vi "Autonomous Independent.vi"() -> ()   [LabVIEW 2019]
doc: "This VI is called when autonomous begins, and will automatically be terminated when autonomous ends. You can carry out timed or sensor driven robot movement independently without needing to return to the caller."
uses:
  <vilib>/Rock Robotics/SystemInterfaces/spilib/spi_bus.ctl
  <vilib>/Rock Robotics/WPI/Utilities/WPI_GetSetVariantRefNum.vi
  <vilib>/Rock Robotics/Network Tables/NT Write Numeric Array.vi
  <vilib>/Rock Robotics/WPI/RobotDrive/WPI_RobotDriveArcadeDrive_Standard(NoSaturation).vi
  <vilib>/Rock Robotics/WPI/Gyro/WPI_GyroXRS450_SPI_Open.vi
  <vilib>/Rock Robotics/Network Tables/NT Write Number.vi
  <vilib>/Rock Robotics/Network Tables/NT Read String.vi
panel:
  out "Ultrasonic 2":dbl
  out "Ultrasonic":dbl
  out "Degrees 2":dbl(knob) scale=0.0..360.0
  out "Degrees":dbl(knob) scale=0.0..360.0
  in  "Reset Angle?":bool
  out "Calibrated?":bool
  out "Degrees":dbl(knob) scale=0.0..360.0
  out "Degrees 2":dbl(knob) scale=0.0..360.0
  in  "SPI Bus":T1
  out "Device Found":bool
  in  "Sample Rate (Hz)":dbl=1000.0 min=50.0 max=20000.0 format="%#_13g"
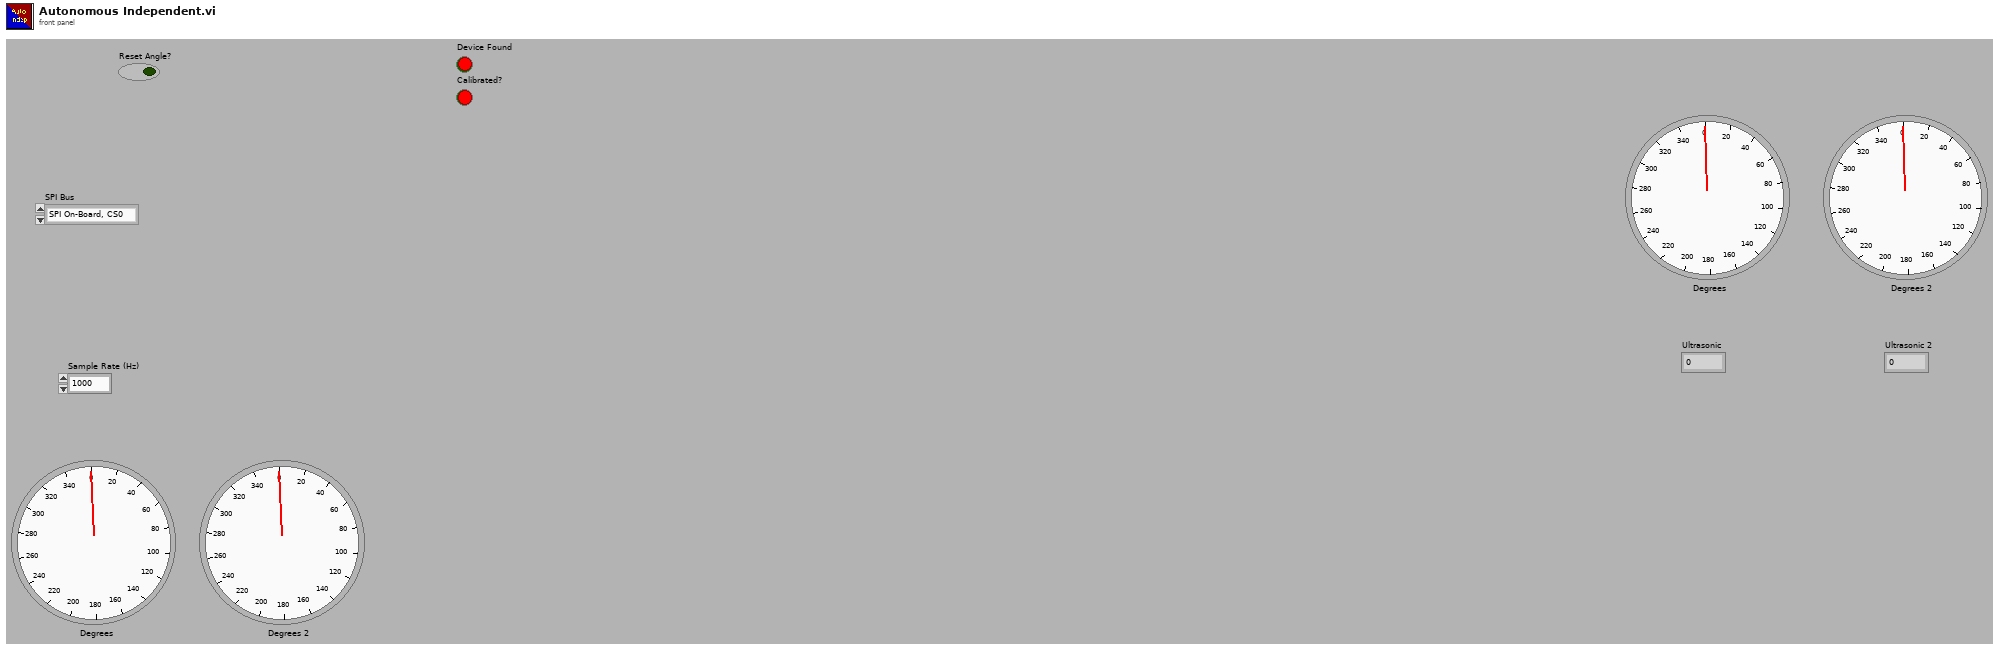
[diagram p1: front panel]
types:
  T1 = typedef "spi_bus.ctl" = enum16{"SPI On-Board, CS0", "SPI On-Board, CS1", "SPI On-Board, CS2", "SPI On-Board, CS3", "SPI MXP", "Invalid"}
  T2 = typedef "WPI_JoystickDevRef.ctl" = cluster{"Device":T3}
  T3 = typedef "WPI_JoystickDeviceEnum.ctl" = enum16{"USB 0", "USB 1", "USB 2", "USB 3", "USB 4", "USB 5"}
  T4 = typedef "WPI_RobotDriveDevRef.ctl" = cluster{"DevStatus":errorcluster, "Motors[]":T5[], "Square Inputs":bool, "Max Output":dbl}
  T5 = typedef "WPI_MotorControlDeviceRef.ctl" = cluster{"DeviceStatus":errorcluster, "Type":T6, "PWM":cluster{"PWM Channel":T7, "DeadBand":T8}, "CAN":cluster{"Device Number":u8, "SetOutput VI Ref":variant, "GetOutput VI Ref":variant, "Enable VI Ref":variant, "Disable VI Ref":variant, "Data":variant}, "Invert":bool, "DIO PWM":cluster{"PWM \"Enable\" Channel":T7, "DIOChannel":T9, "PWM Rate":dbl}}
  T6 = typedef "WPI_MotorControlType.ctl" = enum16{"PWM", "CAN", "DIO PWM"}
  T7 = typedef "FPGA_DIOPWMChannel.ctl" = enum8{"PWM 0", "PWM 1", "PWM 2", "PWM 3", "PWM 4", "PWM 5", "PWM 6", "PWM 7", "PWM 8", "PWM 9", "PWM MXP 0", "PWM MXP 1", "PWM MXP 2", "PWM MXP 3", "PWM MXP 4", "PWM MXP 5", "PWM MXP 6", "PWM MXP 7", "PWM MXP 8", "PWM MXP 9", "Invalid"}
  T8 = typedef "WPI_PWMDeadband.ctl" = cluster{"Name":string, "maxPositivePwm":i32, "minPositivePwm":i32, "centerPwm":i32, "maxNegativePwm":i32, "minNegativePwm":i32, "angularRange":u16}
  T9 = typedef "FPGA_DIOChannel.ctl" = enum8{"DIO 0", "DIO 1", "DIO 2", "DIO 3", "DIO 4", "DIO 5", "DIO 6", "DIO 7", "DIO 8", "DIO 9", "DIO MXP 0", "DIO MXP 1", "DIO MXP 2", "DIO MXP 3", "DIO MXP 4", "DIO MXP 5", "DIO MXP 6", "DIO MXP 7", "DIO MXP 8", "DIO MXP 9", "DIO MXP 10", "DIO MXP 11", "DIO MXP 12", "DIO MXP 13", "DIO MXP 14", "DIO MXP 15", "SPI Port CS1", "SPI Port CS2", "SPI Port CS3", "SPI Port MISO", "SPI Port MOSI", "Invalid"}
  T10 = typedef "WPI_GyroDevRef.ctl" = cluster{"DevStatus":errorcluster, "Analog Channel":T11, "Gain (VoltsPerDegree/Second)":dbl, "Gyro Type":enum16{"Analog", "XRS450"}, "Handle":i32, "SPI Bus":T1, "Device Found":bool, "Sample Rate":dbl, "Calibrate On Open":bool, "Offset":dbl}
  T11 = typedef "FPGA_AIChannel.ctl" = enum8{"AI 0", "AI 1", "AI 2", "AI 3", "AI MXP 0", "AI MXP 1", "AI MXP 2", "AI MXP 3", "Invalid"}
  T12 = typedef "WPI_AnalogChannelDevRef.ctl" = cluster{"DevStatus":errorcluster, "Analog Channel":T11}
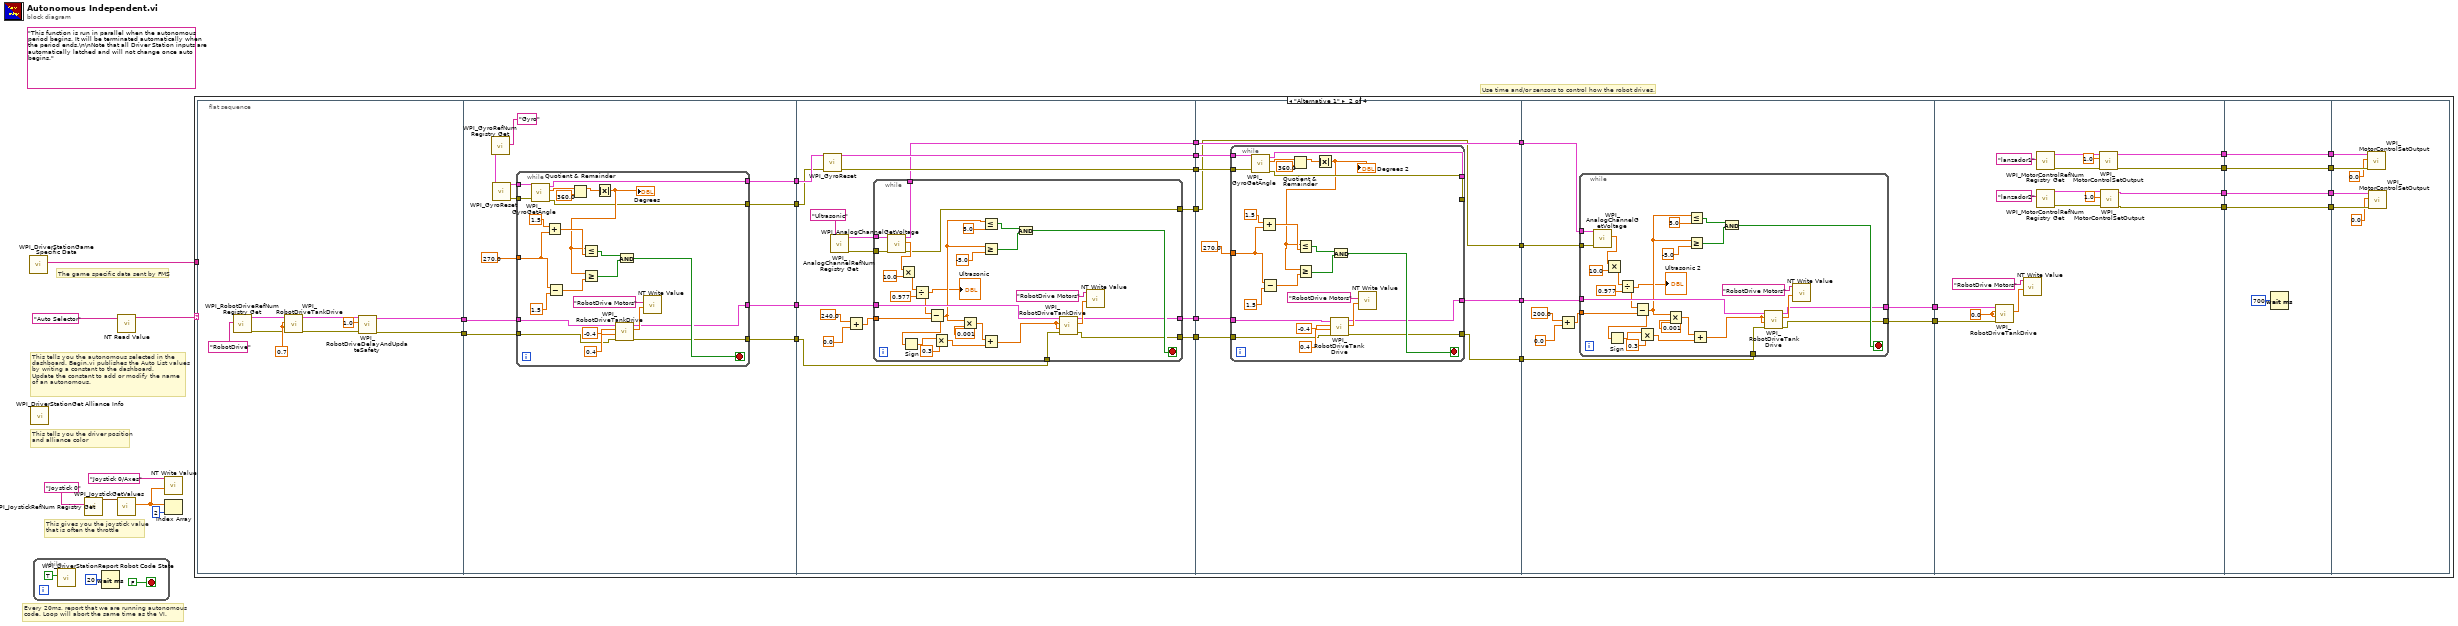
[diagram p0: block diagram]
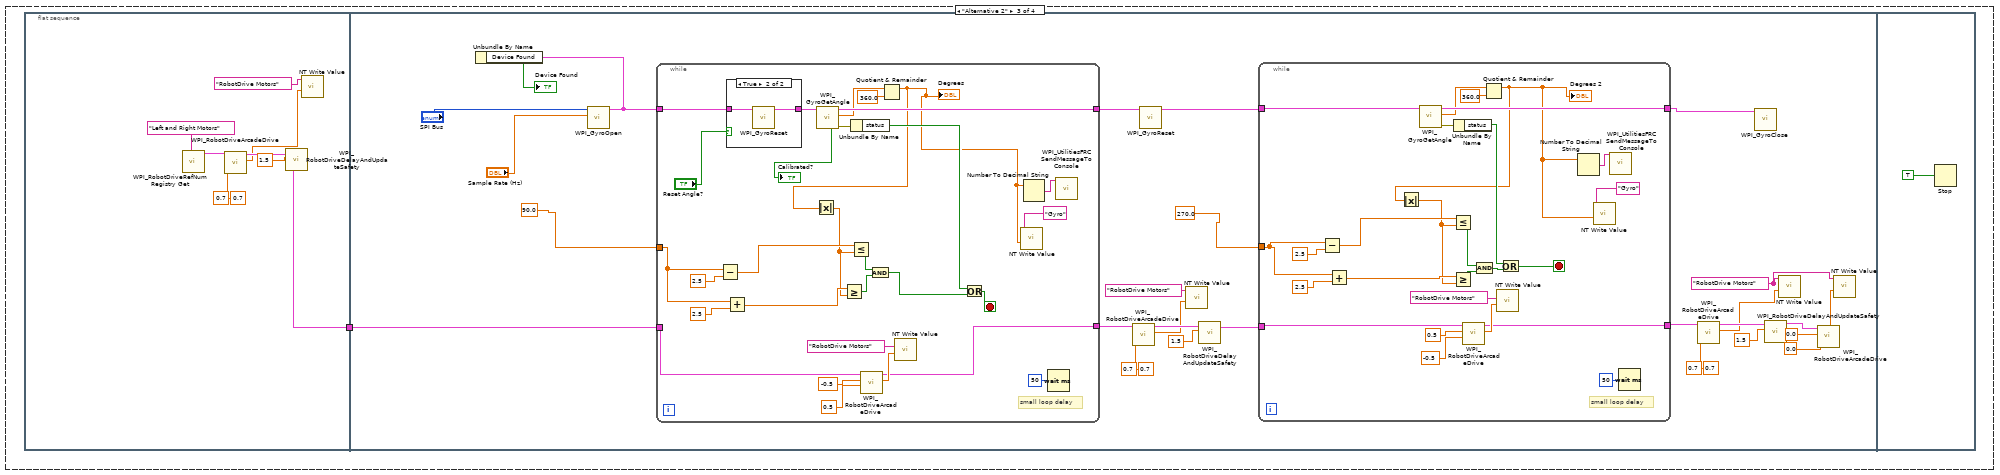
[diagram p3: hidden frame]
diagram:
  (unwired) "This function is run in parallel when the autonomous period begins. It will be terminated automatically when the period ends.\n\nNote that all Driver Station inputs are automatically latched and will not change once auto begins."
  # "The game specific data sent by FMS"
  # "This tells you the autonomous selected in the \ndashboard. Begin.vi publishes the Auto List values\nby writing a constant to the dashboard.\nUpdate the constant to add or modify the name\nof an autonomous."
  # "Every 20ms, report that we are running autonomous\ncode. Loop will abort the same time as the VI."
  # "This gives you the joystick value\nthat is often the throttle"
  # "Use time and/or sensors to control how the robot drives."
  # "This tells you the driver position\nand alliance color"
  n1 = call <vilib>:"WPI_DriverStationGame Specific Data.vi"() -> ("Game Specific Data"=w1:string)  [unwired: 11 in]
  n2 = call <vilib>:"WPI_DriverStationGet Alliance Info.vi"() -> ()  [unwired: 12 out]
  n3 = while {
    stop <- FALSE stop-if-true
    n4 = call <vilib>:"WPI_DriverStationReport Robot Code State.vi"("Autonomous"=TRUE) -> ()  [unwired: 10 in, 1 out]
    n5 = Wait (ms)(milliseconds to wait=u32 20) -> ()  [unwired: 1 out]
  }
  n6 = call <vilib>:"WPI_JoystickRefNum Registry Get.vi"("refnum name"="Joystick 0") -> ("JoystickDevRef"=w7:T2)  [unwired: 1 in, 9 out]
  n7 = call <vilib>:"WPI_JoystickGetValues.vi"("JoystickDevRef"=w7) -> ("Axes"=w3:dbl[])  [unwired: 6 in, 4 out]
  n8 = call-poly <vilib>:"NT Read Value.vi"("Name"="Auto Selector") -> ("String"=w4:string)  [unwired: 9 in, 1 out]
  n9 = call-poly <vilib>:"NT Write Value.vi"("Numeric Array"=w3, "Name"="Joystick 0/Axes") -> ()  [unwired: 9 in, 1 out]
  n10 = Index Array(array=w3, index=2) -> ()  [unwired: 1 out]
  n11 = case shown="\"Alternative 1\"" w4 {
    tunnel: w1 -> [_ _ _ _]
    frame Default {
      # "You can put your main auto here, or you can right-click on the case and make any\nother frame be the default case."
      # "This is the frame that will execute if no selection is made, or if it is not recognized"
    }
    frame "Alternative 1" {
      n12 = flat-sequence {
        tunnel: [w44] -> w13
        tunnel: [w45] -> w12
        tunnel: [w52] -> w37
        tunnel: [w51] -> w36
        tunnel: [w50] -> w35
        tunnel: [w49] -> w34
        tunnel: w13 -> [w48]
        tunnel: w12 -> [w47]
        tunnel: w37 -> [w92]
        tunnel: w36 -> [w91]
        tunnel: w35 -> [w90]
        tunnel: w34 -> [w89]
        tunnel: [w88] -> w33
        tunnel: [w87] -> w32
        tunnel: [w86] -> w31
        tunnel: [w85] -> w30
        tunnel: [w84] -> w26
        tunnel: [w83] -> w24
        tunnel: w33 -> [w135]
        tunnel: w32 -> [w134]
        tunnel: w31 -> [w132]
        tunnel: w30 -> [w131]
        tunnel: [w130] -> w29
        tunnel: [w129] -> w28
        tunnel: [w128] -> w27
        tunnel: w26 -> [w128]
        tunnel: [w127] -> w25
        tunnel: w24 -> [w127]
        tunnel: w29 -> [w168]
        tunnel: w28 -> [w164]
        tunnel: w27 -> [w163]
        tunnel: w25 -> [w162]
        tunnel: [w161] -> w23
        tunnel: [w160] -> w22
        tunnel: w23 -> [w201]
        tunnel: w22 -> [w200]
        tunnel: [w198] -> w20
        tunnel: [w197] -> w18
        tunnel: [w196] -> w16
        tunnel: [w195] -> w14
        tunnel: [w215] -> w21
        tunnel: w20 -> [w215]
        tunnel: [w214] -> w19
        tunnel: w18 -> [w214]
        tunnel: [w213] -> w17
        tunnel: w16 -> [w213]
        tunnel: [w212] -> w15
        tunnel: w14 -> [w212]
        tunnel: w21 -> [w222]
        tunnel: w19 -> [w221]
        tunnel: w17 -> [w220]
        tunnel: w15 -> [w219]
        frame #0 {
          w40 = 0.7 ("Left axis value")
          n13 = call <vilib>:"WPI_RobotDriveRefNum Registry Get.vi"("refnum name"="RobotDrive") -> ("error out"=w38:errorcluster, "RobotDriveDevRef"=w39:T4)  [unwired: 9 in]
          n14 = call <vilib>:"WPI_RobotDriveTankDrive.vi"("error in (no error)"=w38, "Right axis value"=w40, "Left axis value"=w40, "RobotDriveDevRef"=w39) -> ("error out"=w41:errorcluster, "RobotDriveDevRef"=w42:T4)  [unwired: 5 in, 1 out]
          n15 = call <vilib>:"WPI_RobotDriveDelayAndUpdateSafety.vi"("error in (no error)"=w41, "Delay (s)"=1.0, "RobotDriveDevRef"=w42) -> ("error out"=w44:errorcluster, "RobotDriveDevRef 2"=w45:T4)  [unwired: 7 in]
        }
        frame #1 {
          n16 = call <vilib>:"WPI_GyroRefNum Registry Get.vi"("refnum name"="Gyro") -> ("error out"=w56:errorcluster, "GyroDevRef"=w57:T10)  [unwired: 9 in]
          n17 = call <vilib>:"WPI_GyroReset.vi"("error in"=w56, "GyroDevRef"=w57) -> ("error out"=w54:errorcluster, "GyroDevRef"=w55:T10)  [unwired: 8 in]
          n18 = while {
            tunnel: w55 -> [w82]
            tunnel: w54 -> [w81]
            tunnel: 270.0 ("y") -> [w73]
            tunnel: [w64] -> w52
            tunnel: [w63] -> w51
            tunnel: [w62] -> w50
            tunnel: [w61] -> w49
            tunnel: w48 -> [w60]
            tunnel: w47 -> [w59]
            stop <- w76 stop-if-true
            n19 = call <vilib>:"WPI_GyroGetAngle.vi"("error in"=w81, "GyroDevRef"=w82) -> ("error out"=w61:errorcluster, "Angle"=w68:dbl, "GyroDevRef"=w62:T10)  [unwired: 5 in, 2 out]
            n20 = Add(x=1.5 ("y"), y=w73) -> (x+y=w69:dbl)
            n21 = Subtract(x=w73, y=1.5 ("x")) -> (x-y=w70:dbl)
            n22 = Quotient & Remainder(x=w68, y=360.0) -> (x-y*floor(x/y)=w66:dbl)  [unwired: 1 out]
            n23 = Absolute Value(x=w66) -> (abs(x)=w65:dbl)
            "Degrees" <- w65
            n24 = Less Or Equal?(x=w65, y=w69) -> (x <= y?=w71:bool)
            n25 = Greater Or Equal?(x=w65, y=w70) -> (x >= y?=w72:bool)
            n26 = call <vilib>:"WPI_RobotDriveTankDrive.vi"("error in (no error)"=w60, "Right axis value"=0.4 ("X axis value"), "Left axis value"=-0.4 ("X axis value"), "RobotDriveDevRef"=w59) -> ("error out"=w63:errorcluster, "Motor Values"=w80:dbl[], "RobotDriveDevRef"=w64:T4)  [unwired: 5 in]
            n27 = And(x=w71, y=w72) -> (x .and. y?=w76:bool)
            n28 = call-poly <vilib>:"NT Write Value.vi"("Numeric Array"=w80, "Name"="RobotDrive Motors") -> ()  [unwired: 9 in, 1 out]
          }
        }
        frame #2 {
          n29 = call <vilib>:"WPI_GyroReset.vi"("error in"=w89, "GyroDevRef"=w90) -> ("error out"=w85:errorcluster, "GyroDevRef"=w86:T10)  [unwired: 8 in]
          n30 = call <vilib>:"WPI_AnalogChannelRefNum Registry Get.vi"("refnum name"="Ultrasonic") -> ("error out"=w97:errorcluster, "AIDeviceRef"=w96:T12)  [unwired: 9 in]
          n31 = Add(x=240.0 ("y"), y=0.0) -> (x+y=w93:dbl)
          n32 = while {
            tunnel: w97 -> [w122]
            tunnel: w96 -> [w121]
            tunnel: w93 -> [w120]
            tunnel: w92 -> [w115]
            tunnel: w91 -> [w111]
            tunnel: [w103] -> w88
            tunnel: [w102] -> w87
            tunnel: [w100] -> w84
            tunnel: [w99] -> w83
            stop <- w107 stop-if-true
            n33 = call <vilib>:"WPI_AnalogChannelGetVoltage.vi"("error in (no error)"=w122, "AIDeviceRef"=w121) -> ("error out"=w99:errorcluster, "Voltage"=w125:dbl, "AIDeviceRef"=w100:T12)  [unwired: 7 in]
            n34 = Multiply(x=w125, y=10.0) -> (x*y=w126:dbl)
            n35 = Divide(x=w126, y=0.977) -> (x/y=w101:dbl)
            "Ultrasonic" <- w101
            n36 = Subtract(x=w101, y=w120) -> (x-y=w104:dbl)
            n37 = Sign(1:w104) -> (0:w114:dbl)
            n38 = Multiply(x=w114, y=0.3) -> (x*y=w112:dbl)
            n39 = Multiply(x=w104, y=0.001) -> (x*y=w118:dbl)
            n40 = Less Or Equal?(x=w104, y=5.0 ("x")) -> (x <= y?=w109:bool)
            n41 = Greater Or Equal?(x=w104, y=-5.0 ("x")) -> (x >= y?=w108:bool)
            n42 = Add(x=w118, y=w112) -> (x+y=w110:dbl)
            n43 = And(x=w109, y=w108) -> (x .and. y?=w107:bool)
            n44 = call <vilib>:"WPI_RobotDriveTankDrive.vi"("error in (no error)"=w111, "Right axis value"=w110, "Left axis value"=w110, "RobotDriveDevRef"=w115) -> ("error out"=w103:errorcluster, "Motor Values"=w117:dbl[], "RobotDriveDevRef"=w102:T4)  [unwired: 5 in]
            n45 = call-poly <vilib>:"NT Write Value.vi"("Numeric Array"=w117, "Name"="RobotDrive Motors") -> ()  [unwired: 9 in, 1 out]
          }
        }
        frame #3 {
          n46 = while {
            tunnel: w134 -> [w155]
            tunnel: w135 -> [w154]
            tunnel: 270.0 ("y") -> [w150]
            tunnel: [w142] -> w130
            tunnel: [w141] -> w129
            tunnel: [w140] -> _
            tunnel: [w139] -> _
            tunnel: w132 -> [w136]
            tunnel: w131 -> [w137]
            stop <- w153 stop-if-true
            n47 = call <vilib>:"WPI_GyroGetAngle.vi"("error in"=w137, "GyroDevRef"=w136) -> ("error out"=w139:errorcluster, "Angle"=w145:dbl, "GyroDevRef"=w140:T10)  [unwired: 5 in, 2 out]
            n48 = Add(x=1.5 ("y"), y=w150) -> (x+y=w146:dbl)
            n49 = Subtract(x=w150, y=1.5 ("x")) -> (x-y=w147:dbl)
            n50 = Quotient & Remainder(x=w145, y=360.0) -> (x-y*floor(x/y)=w143:dbl)  [unwired: 1 out]
            n51 = Absolute Value(x=w143) -> (abs(x)=w138:dbl)
            "Degrees 2" <- w138
            n52 = Less Or Equal?(x=w138, y=w146) -> (x <= y?=w148:bool)
            n53 = Greater Or Equal?(x=w138, y=w147) -> (x >= y?=w149:bool)
            n54 = call <vilib>:"WPI_RobotDriveTankDrive.vi"("error in (no error)"=w154, "Right axis value"=0.4 ("X axis value"), "Left axis value"=-0.4 ("X axis value"), "RobotDriveDevRef"=w155) -> ("error out"=w141:errorcluster, "Motor Values"=w159:dbl[], "RobotDriveDevRef"=w142:T4)  [unwired: 5 in]
            n55 = And(x=w148, y=w149) -> (x .and. y?=w153:bool)
            n56 = call-poly <vilib>:"NT Write Value.vi"("Numeric Array"=w159, "Name"="RobotDrive Motors") -> ()  [unwired: 9 in, 1 out]
          }
        }
        frame #4 {
          n57 = Add(x=200.0 ("y"), y=0.0) -> (x+y=w165:dbl)
          n58 = while {
            tunnel: w162 -> [w190]
            tunnel: w163 -> [w189]
            tunnel: w165 -> [w188]
            tunnel: w168 -> [w183]
            tunnel: w164 -> [w179]
            tunnel: [w170] -> w161
            tunnel: [w169] -> w160
            stop <- w175 stop-if-true
            n59 = call <vilib>:"WPI_AnalogChannelGetVoltage.vi"("error in (no error)"=w190, "AIDeviceRef"=w189) -> ("Voltage"=w193:dbl)  [unwired: 7 in, 2 out]
            n60 = Multiply(x=w193, y=10.0) -> (x*y=w194:dbl)
            n61 = Divide(x=w194, y=0.977) -> (x/y=w171:dbl)
            "Ultrasonic 2" <- w171
            n62 = Subtract(x=w171, y=w188) -> (x-y=w172:dbl)
            n63 = Sign(1:w172) -> (0:w182:dbl)
            n64 = Multiply(x=w182, y=0.3) -> (x*y=w180:dbl)
            n65 = Multiply(x=w172, y=0.001) -> (x*y=w186:dbl)
            n66 = Less Or Equal?(x=w172, y=5.0 ("x")) -> (x <= y?=w177:bool)
            n67 = Greater Or Equal?(x=w172, y=-5.0 ("x")) -> (x >= y?=w176:bool)
            n68 = Add(x=w186, y=w180) -> (x+y=w178:dbl)
            n69 = And(x=w177, y=w176) -> (x .and. y?=w175:bool)
            n70 = call <vilib>:"WPI_RobotDriveTankDrive.vi"("error in (no error)"=w179, "Right axis value"=w178, "Left axis value"=w178, "RobotDriveDevRef"=w183) -> ("error out"=w169:errorcluster, "Motor Values"=w185:dbl[], "RobotDriveDevRef"=w170:T4)  [unwired: 5 in]
            n71 = call-poly <vilib>:"NT Write Value.vi"("Numeric Array"=w185, "Name"="RobotDrive Motors") -> ()  [unwired: 9 in, 1 out]
          }
        }
        frame #5 {
          w199 = 0.0 ("Left axis value")
          n72 = call <vilib>:"WPI_RobotDriveTankDrive.vi"("error in (no error)"=w200, "Right axis value"=w199, "Left axis value"=w199, "RobotDriveDevRef"=w201) -> ("Motor Values"=w203:dbl[])  [unwired: 5 in, 2 out]
          n73 = call-poly <vilib>:"NT Write Value.vi"("Numeric Array"=w203, "Name"="RobotDrive Motors") -> ()  [unwired: 9 in, 1 out]
          n74 = call <vilib>:"WPI_MotorControlRefNum Registry Get.vi"("refnum name"="lanzador1") -> ("error out"=w210:errorcluster, "MotorControlDevRef"=w211:T5)  [unwired: 9 in]
          n75 = call <vilib>:"WPI_MotorControlRefNum Registry Get.vi"("refnum name"="lanzador2") -> ("error out"=w206:errorcluster, "MotorControlDevRef"=w207:T5)  [unwired: 9 in]
          n76 = call <vilib>:"WPI_MotorControlSetOutput.vi"("error in (no error)"=w210, "Output"=1.0, "MotorControlDevRef"=w211) -> ("error out"=w195:errorcluster, "MotorControlDevRef"=w198:T5)  [unwired: 6 in, 1 out]
          n77 = call <vilib>:"WPI_MotorControlSetOutput.vi"("error in (no error)"=w206, "Output"=1.0, "MotorControlDevRef"=w207) -> ("error out"=w196:errorcluster, "MotorControlDevRef"=w197:T5)  [unwired: 6 in, 1 out]
        }
        frame #6 {
          n78 = Wait (ms)(milliseconds to wait=u32 700) -> ()  [unwired: 1 out]
        }
        frame #7 {
          n79 = call <vilib>:"WPI_MotorControlSetOutput.vi"("error in (no error)"=w219, "Output"=0.0, "MotorControlDevRef"=w222) -> ()  [unwired: 6 in, 3 out]
          n80 = call <vilib>:"WPI_MotorControlSetOutput.vi"("error in (no error)"=w220, "Output"=0.0, "MotorControlDevRef"=w221) -> ()  [unwired: 6 in, 3 out]
        }
      }
    }
    frame "Alternative 2" {
      n81 = flat-sequence {
        tunnel: [w231] -> w223
        tunnel: w223 -> [w260]
        frame #0 {
          n82 = call <vilib>:"WPI_RobotDriveRefNum Registry Get.vi"("refnum name"="Left and Right Motors") -> ("RobotDriveDevRef"=w229:T4)  [unwired: 1 in, 9 out]
          n83 = call-poly <vilib>:"WPI_RobotDriveArcadeDrive.vi"("Y axis value"=0.7, "X axis value"=0.7, "RobotDriveDevRef"=w229) -> ("Motor Values"=w225:dbl[], "RobotDriveDevRef"=w228:T4)  [unwired: 1 in, 6 out]
          n84 = call <vilib>:"WPI_RobotDriveDelayAndUpdateSafety.vi"("Delay (s)"=1.5, "RobotDriveDevRef"=w228) -> ("RobotDriveDevRef 2"=w231:T4)  [unwired: 8 in, 1 out]
          n85 = call-poly <vilib>:"NT Write Value.vi"("Numeric Array"=w225, "Name"="RobotDrive Motors") -> ()  [unwired: 9 in, 1 out]
        }
        frame #1 {
          w242 = "RobotDrive Motors" ("Name")
          n86 = call-poly <vilib>:"WPI_GyroOpen.vi"("Sample Rate (Hz)"="Sample Rate (Hz)", "SPI Bus"="SPI Bus") -> ("GyroDevRef"=w261:T10)  [unwired: 7 in, 2 out]
          n87 = Unbundle By Name(w261) -> ("Device Found"=→"Device Found":bool)
          n88 = while {
            tunnel: w261 -> [w314]
            tunnel: [w312] -> w254
            tunnel: 90.0 ("Angle 3") -> [w296]
            tunnel: w260 -> [w304]
            tunnel: [w303] -> w255
            stop <- w309 stop-if-true
            # "small loop delay"
            n89 = Subtract(x=w296, y=2.5) -> (x-y=w298:dbl)
            n90 = case shown="True" "Reset Angle?" {
              tunnel: w314 -> [w317 w319]
              tunnel: [w317 w318] -> w313
              frame False {
              }
              frame True {
                n91 = call <vilib>:"WPI_GyroReset.vi"("GyroDevRef"=w319) -> ("GyroDevRef"=w318:T10)  [unwired: 9 in, 1 out]
              }
            }
            n92 = Add(x=w296, y=2.5) -> (x+y=w295:dbl)
            n93 = call <vilib>:"WPI_GyroGetAngle.vi"("GyroDevRef"=w313) -> ("error out"=w310:errorcluster, "Angle"=w311:dbl, "GyroDevRef"=w312:T10, "Calibrated?"=→"Calibrated?":bool)  [unwired: 6 in, 1 out]
            n94 = Unbundle By Name(w310) -> ("status"=w302:bool)
            n95 = call-poly <vilib>:"WPI_RobotDriveArcadeDrive.vi"("Y axis value"=0.5 ("X axis value"), "X axis value"=-0.5, "RobotDriveDevRef"=w304) -> ("Motor Values"=w308:dbl[], "RobotDriveDevRef"=w303:T4)  [unwired: 1 in, 6 out]
            n96 = Quotient & Remainder(x=w311, y=360.0) -> (x-y*floor(x/y)=w288:dbl)  [unwired: 1 out]
            "Degrees" <- w288
            n97 = Absolute Value(x=w288) -> (abs(x)=w294:dbl)
            n98 = Greater Or Equal?(x=w295, y=w294) -> (x >= y?=w292:bool)
            n99 = Less Or Equal?(x=w298, y=w294) -> (x <= y?=w293:bool)
            n100 = And(x=w293, y=w292) -> (x .and. y?=w291:bool)
            n101 = call-poly <vilib>:"NT Write Value.vi"("Numeric Array"=w308, "Name"="RobotDrive Motors") -> ()  [unwired: 9 in, 1 out]
            n102 = Or(x=w302, y=w291) -> (x .or. y?=w309:bool)
            n103 = call-poly <vilib>:"NT Write Value.vi"("Numeric"=w288, "Name"="Gyro") -> ()  [unwired: 9 in, 1 out]
            n104 = Number To Decimal String(number=w288) -> (decimal integer string=w289:string)  [unwired: 1 in]
            n105 = Wait (ms)(milliseconds to wait=u32 50) -> ()  [unwired: 1 out]
            n106 = call <vilib>:"WPI_UtilitiesFRC SendMessageToConsole.vi"("Message"=w289) -> ()  [unwired: 14 in, 1 out]
          }
          n107 = call-poly <vilib>:"WPI_RobotDriveArcadeDrive.vi"("Y axis value"=0.7, "X axis value"=0.7, "RobotDriveDevRef"=w255) -> ("Motor Values"=w245:dbl[], "RobotDriveDevRef"=w258:T4)  [unwired: 1 in, 6 out]
          n108 = call <vilib>:"WPI_GyroReset.vi"("GyroDevRef"=w254) -> ("GyroDevRef"=w253:T10)  [unwired: 9 in, 1 out]
          n109 = call-poly <vilib>:"NT Write Value.vi"("Numeric Array"=w245, "Name"="RobotDrive Motors") -> ()  [unwired: 9 in, 1 out]
          n110 = call <vilib>:"WPI_RobotDriveDelayAndUpdateSafety.vi"("Delay (s)"=1.5, "RobotDriveDevRef"=w258) -> ("RobotDriveDevRef 2"=w252:T4)  [unwired: 8 in, 1 out]
          n111 = while {
            tunnel: w253 -> [w274]
            tunnel: [w285] -> w238
            tunnel: 270.0 ("Angle 4") -> [w270]
            tunnel: w252 -> [w277]
            tunnel: [w276] -> w247
            stop <- w282 stop-if-true
            # "small loop delay"
            n112 = Subtract(x=w270, y=2.5) -> (x-y=w272:dbl)
            n113 = Add(x=w270, y=2.5) -> (x+y=w271:dbl)
            n114 = call <vilib>:"WPI_GyroGetAngle.vi"("GyroDevRef"=w274) -> ("error out"=w283:errorcluster, "Angle"=w284:dbl, "GyroDevRef"=w285:T10)  [unwired: 6 in, 2 out]
            n115 = Unbundle By Name(w283) -> ("status"=w275:bool)
            n116 = call-poly <vilib>:"WPI_RobotDriveArcadeDrive.vi"("Y axis value"=-0.5 ("X axis value"), "X axis value"=0.5, "RobotDriveDevRef"=w277) -> ("Motor Values"=w281:dbl[], "RobotDriveDevRef"=w276:T4)  [unwired: 1 in, 6 out]
            n117 = Quotient & Remainder(x=w284, y=360.0) -> (x-y*floor(x/y)=w262:dbl)  [unwired: 1 out]
            "Degrees 2" <- w262
            n118 = Absolute Value(x=w262) -> (abs(x)=w268:dbl)
            n119 = Less Or Equal?(x=w272, y=w268) -> (x <= y?=w267:bool)
            n120 = Greater Or Equal?(x=w271, y=w268) -> (x >= y?=w266:bool)
            n121 = And(x=w267, y=w266) -> (x .and. y?=w265:bool)
            n122 = call-poly <vilib>:"NT Write Value.vi"("Numeric Array"=w281, "Name"="RobotDrive Motors") -> ()  [unwired: 9 in, 1 out]
            n123 = Or(x=w275, y=w265) -> (x .or. y?=w282:bool)
            n124 = Number To Decimal String(number=w262) -> (decimal integer string=w263:string)  [unwired: 1 in]
            n125 = call-poly <vilib>:"NT Write Value.vi"("Numeric"=w262, "Name"="Gyro") -> ()  [unwired: 9 in, 1 out]
            n126 = call <vilib>:"WPI_UtilitiesFRC SendMessageToConsole.vi"("Message"=w263) -> ()  [unwired: 14 in, 1 out]
            n127 = Wait (ms)(milliseconds to wait=u32 50) -> ()  [unwired: 1 out]
          }
          n128 = call-poly <vilib>:"WPI_RobotDriveArcadeDrive.vi"("Y axis value"=0.7, "X axis value"=0.7, "RobotDriveDevRef"=w247) -> ("Motor Values"=w243:dbl[], "RobotDriveDevRef"=w250:T4)  [unwired: 1 in, 6 out]
          n129 = call <vilib>:"WPI_GyroClose.vi"("GyroDevRef"=w238) -> ()  [unwired: 10 in, 1 out]
          n130 = call <vilib>:"WPI_RobotDriveDelayAndUpdateSafety.vi"("Delay (s)"=1.5, "RobotDriveDevRef"=w250) -> ("RobotDriveDevRef 2"=w246:T4)  [unwired: 8 in, 1 out]
          n131 = call-poly <vilib>:"NT Write Value.vi"("Numeric Array"=w243, "Name"=w242) -> ()  [unwired: 9 in, 1 out]
          n132 = call-poly <vilib>:"WPI_RobotDriveArcadeDrive.vi"("Y axis value"=0.0, "X axis value"=0.0, "RobotDriveDevRef"=w246) -> ("Motor Values"=w241:dbl[])  [unwired: 1 in, 7 out]
          n133 = call-poly <vilib>:"NT Write Value.vi"("Numeric Array"=w241, "Name"=w242) -> ()  [unwired: 9 in, 1 out]
        }
        frame #2 {
          n134 = Stop(stop? (T)=TRUE) -> ()
        }
      }
    }
    frame "Stellar" {
    }
  }
